vi "FL_Preprocess_and_save_incrementally.vi"(0 "Temporary file output path":path, 1 "Loop iteration":i32, 2 "Mouse face dir. swap":bool, 3 "Loop speed in ms":u16, 4 "Save every N seconds":u32=15, 5 "error in (no error)":errorcluster, 6 "Filter type":u16(ring)=5 items=["None", "Kalman 0.50", "Kalman 0.30", "Kalman 0.12", "Savitzky-Golay 3/5", "Savitzky-Golay 3/11", "Savitzky-Golay 3/31"], 7 "Sensor read input":T3(array[cluster]), 8 "Offset":sgl, 10 "Pixels per mm":dbl, 11 "Data flow controls in":T2, 12 "Diagram at recording bounds":T1, 13 "Sensor board size":string="Small") -> (14 "Eff. save interval":sgl, 15 "Latest sensor output (decoded)":string[][](array[string]), 16 "Fire TTL":bool, 17 "TTL out N":u8, 18 "Current TTL status":u8, 19 "error out":errorcluster)   [LabVIEW 2016]
uses:
  <vilib>/Utility/miscctls.llb/LVBoundsTypeDef.ctl
  SW_Globals.vi
  <vilib>/Utility/file.llb/Write Delimited Spreadsheet (string).vi
panel:
  in  "Max chunk size":i64=100000
  in  "Number of the file chunk":i32
  out "Chunk size (in bytes)":i64
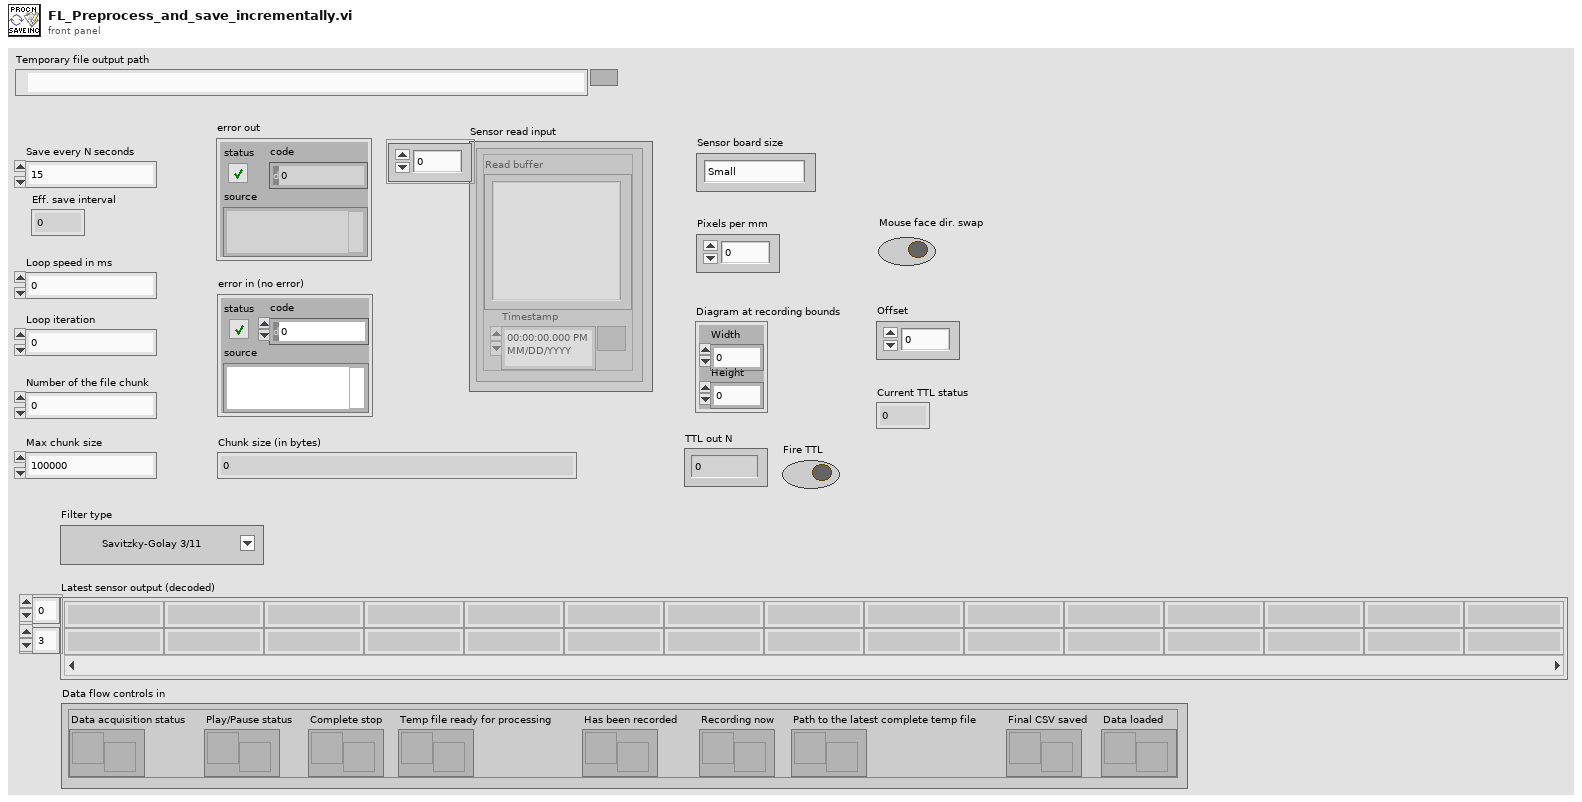
[diagram p1: front panel]
types:
  T1 = typedef "LVBoundsTypeDef.ctl" = cluster{"Width":u32, "Height":u32}
  T2 = cluster{"Data acquisition status":refnum<notifier>, "Play/Pause status":refnum<notifier>, "Complete stop":refnum<notifier>, "Temp file ready for processing":refnum<notifier>, "Has been recorded":refnum<notifier>, "Recording now":refnum<notifier>, "Path to the latest complete temp file":refnum<notifier>, "Final CSV saved":refnum<notifier>, "Data loaded":refnum<notifier>}
  T3 = cluster{"Read buffer":string, "Timestamp":timestamp}[]
  T4 = cluster{"ms since ON":u32, "delta time":u32, "X1":sgl, "Y1":sgl, "X2":sgl, "Y2":sgl, "TTL inputs":u8, "TTL outputs":u8, "Frame timestamp":timestamp, "Frame OK":bool}
  T5 = cluster{"X1 filtered":dbl, "Y1 filtered":dbl, "X2 filtered":dbl, "Y2 filtered":dbl, "X1 raw":dbl, "Y1 raw":dbl, "X2 raw":dbl, "Y2 raw":dbl}
  T6 = cluster{"R from center":dbl, "sin(a)":dbl, "Mouse Xc":dbl, "Mouse Yc":dbl, "X1-X2":dbl, "Y1-Y2":dbl, "Cage Xc":dbl, "Cage Yc":dbl}
  T7 = cluster{"R from center":dbl, "phi (mouse angular position in the cage)":dbl, "alpha (mouse rot. angle)":sgl, "X":dbl, "Y":dbl, "theta (from center towards mouse)":dbl, "beta (cage rot. against mouse)":sgl, "w (mouse angle to wall)":dbl}
  T8 = cluster{"Zone[1]":bool, "Zone[2]":bool, "Zone[3]":bool, "Zone[4]":bool, "Zone[5]":bool, "Zone[6]":bool, "Zone[7]":bool, "Zone[8]":bool, "Zone[9]":bool, "Zone[10]":bool, "Zone[11]":bool, "Zone[12]":bool, "Zone[13]":bool}
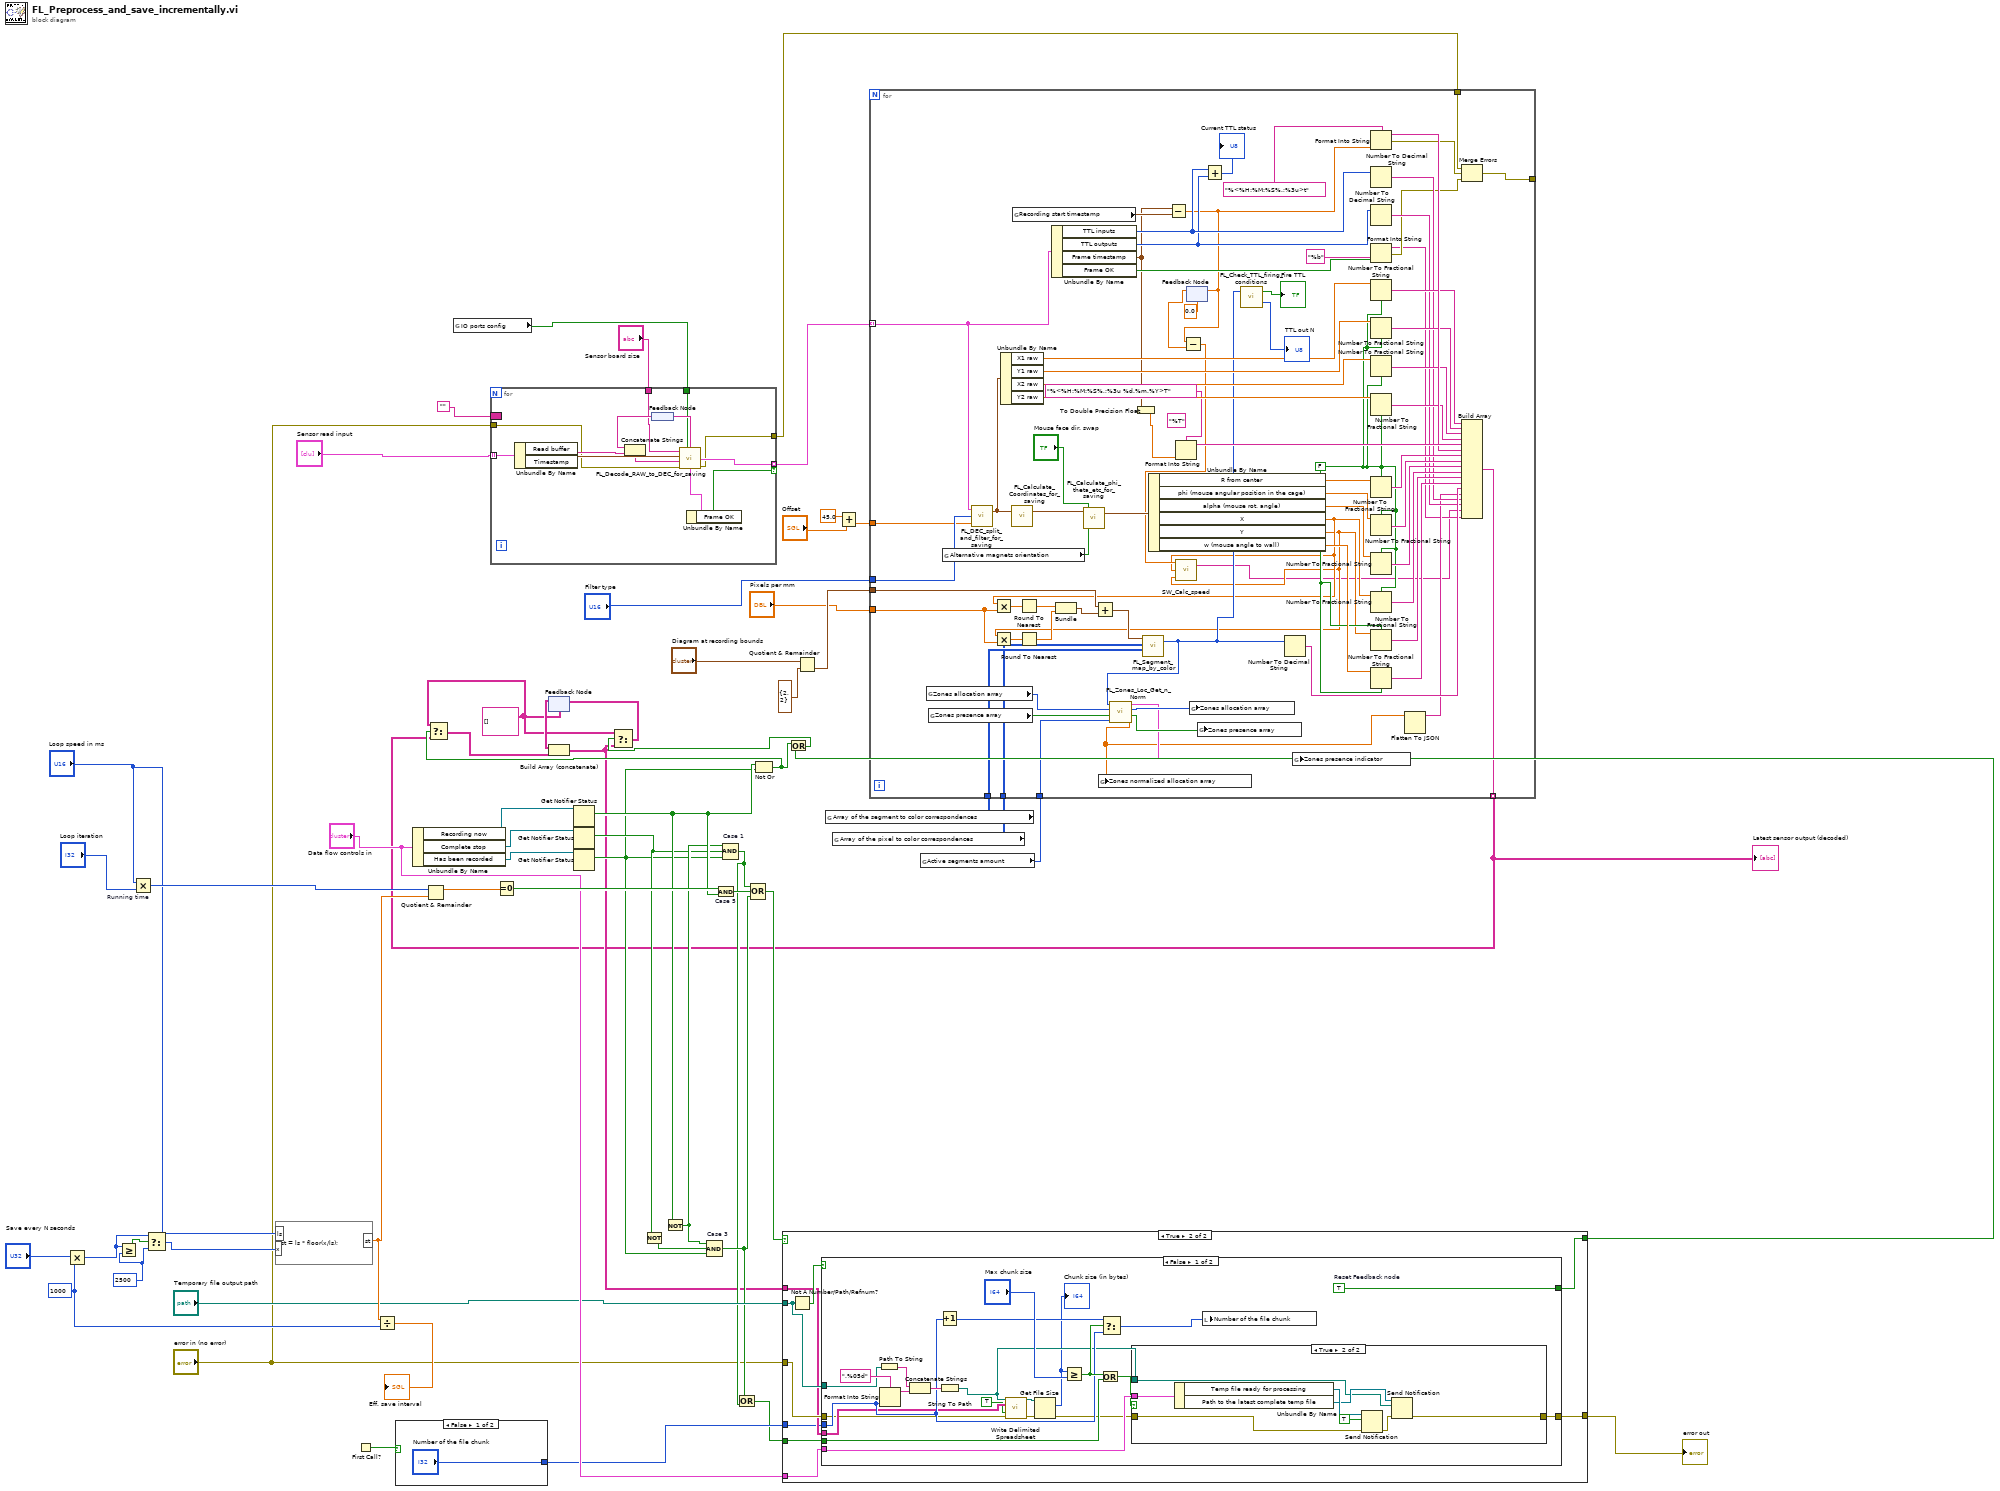
[diagram p0: block diagram]
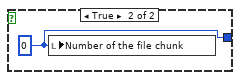
[diagram p2: hidden frame]
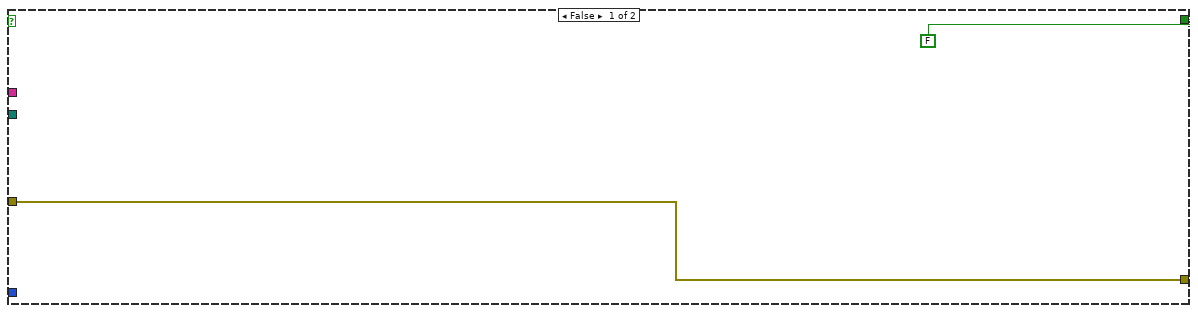
[diagram p3: hidden frame]
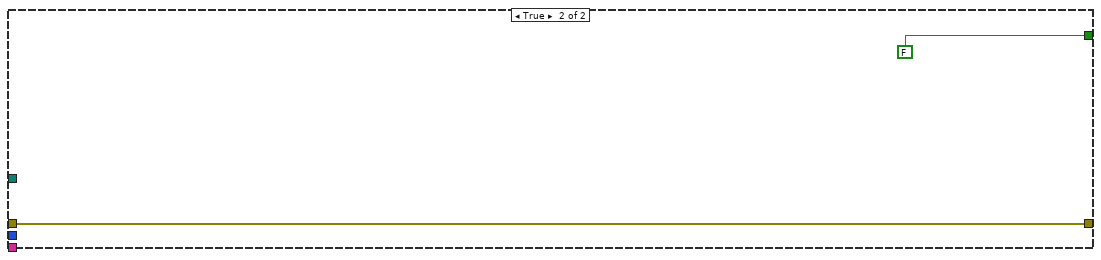
[diagram p5: hidden frame]
diagram:
  w31 = string[][] []
  w45 = u32 1000 ("y")
  w52 = 2500
  n1 = Multiply(x="Save every N seconds", y=w45) -> (x*y=w48:u32)
  n2 = Greater Or Equal?(x=w48, y=w52) -> (x >= y?=w53:bool)
  n3 = Multiply "Running time"(x="Loop speed in ms", y="Loop iteration") -> (x*y=w56:i32)
  n4 = Select(t=w48, s=w53, f=w52) -> (s? t:f=w50:u32)
  n5 = formula code="st = ls * floor(x/ls);"("ls"="Loop speed in ms", "x"=w50) -> ("st"=w47:dbl)
  n6 = First Call?() -> (First Call?: T/F=w40:bool)
  n7 = Divide(x=w47, y=w45) -> (x/y=→"Eff. save interval":dbl)
  n8 = case shown="False" w40 {
    tunnel: ["Number of the file chunk" w60] -> w34
    frame False {
    }
    frame True {
      w60 = 0 ("Number of the file chunk")
      n9 = local write "Number of the file chunk"(w60) -> ()
    }
  }
  n10 = Unbundle By Name("Data flow controls in") -> ("Recording now"=w39:refnum<notifier>, "Complete stop"=w38:refnum<notifier>, "Has been recorded"=w37:refnum<notifier>)
  n11 = Quotient & Remainder(x=w56, y=w47) -> (x-y*floor(x/y)=w54:dbl)  [unwired: 1 out]
  n12 = global read "SW_Globals.vi" "IO ports config"() -> (w1:bool[])
  n13 = for {
    tunnel: "Sensor read input" -> [w72] mode=indexing
    border: "" -> [_]
    tunnel: [w67] -> w18 mode=indexing if=w66
    tunnel: [w64] -> w19
    tunnel: "error in (no error)" -> [w63]
    tunnel: "Sensor board size" -> [w62]
    tunnel: w1 -> [w61]
    n14 = Unbundle By Name(w72) -> ("Read buffer"=w65:string, "Timestamp"=w71:timestamp)
    n15 = feedback #1() -> (w68:string)
    n16 = Concatenate Strings(w68, w65) -> (w70:string)
    n17 = call "FL_Decode_RAW_to_DEC_for_saving.vi"("Sensor board size"=w62, "IO ports config"=w61, "Input timestamp"=w71, "Input string"=w70, "Error In"=w63) -> ("Output string leftover"=w69:string, "DEC output cluster"=w67:T4, "Error Out"=w64:errorcluster)  [unwired: 1 in]
    n18 = feedback-in #1(w69) -> ()
    n19 = Unbundle By Name(w67) -> ("Frame OK"=w66:bool)
  }
  n20 = Equal To 0?(x=w54) -> (x = 0?=w55:bool)
  n21 = feedback #2(w31) -> (w43:string[][])
  n22 = Get Notifier Status(notifier=w39) -> (current notification=w28:bool)  [unwired: 1 in, 4 out]
  n23 = Get Notifier Status(notifier=w38) -> (current notification=w26:bool)  [unwired: 1 in, 4 out]
  n24 = Get Notifier Status(notifier=w37) -> (current notification=w25:bool)  [unwired: 1 in, 4 out]
  n25 = Not(x=w26) -> (.not. x?=w24:bool)
  n26 = Not(x=w28) -> (.not. x?=w27:bool)
  n27 = Compound Arithmetic op=AND "Case 3"(w27, w24, w25) -> (w33:bool)
  n28 = And "Case 5"(x=w55, y=w28) -> (x .and. y?=w58:bool)
  n29 = Compound Arithmetic op=AND "Case 1"(w27, w26, w25) -> (w22:bool)
  n30 = Or(x=w33, y=w22) -> (x .or. y?=w23:bool)
  n31 = Compound Arithmetic op=OR(w22, w58, w33) -> (w44:bool)
  n32 = Not Or(1:w25, 2:w28) -> (0:w30:bool)
  n33 = Quotient & Remainder(x="Diagram at recording bounds", y=T1 {"Width"=2, "Height"=2}) -> (floor(x/y)=w10:T1)  [unwired: 1 out]
  n34 = global read "SW_Globals.vi" "Array of the segment to color correspondences"() -> (w8:u32[][])
  n35 = global read "SW_Globals.vi" "Array of the pixel to color correspondences"() -> (w7:u32[][])
  n36 = Add(x=sgl 45.0, y="Offset") -> (x+y=w3:sgl)
  n37 = global read "SW_Globals.vi" "Active segments amount"() -> (w5:u8)
  n38 = for {
    tunnel: w18 -> [w146] mode=indexing
    tunnel: [w118] -> _
    tunnel: w19 -> [w117]
    tunnel: [w116] -> w16 mode=indexing
    tunnel: "Filter type" -> [w115]
    tunnel: w10 -> [w108]
    tunnel: "Pixels per mm" -> [w114]
    tunnel: w8 -> [w106]
    tunnel: w7 -> [w105]
    tunnel: w5 -> [w101]
    tunnel: w3 -> [w92]
    w120 = FALSE ("use system decimal point (T)")
    (unwired) "%T" ("format string")
    n39 = global read "SW_Globals.vi" "Zones allocation array"() -> (w102:i32[])
    n40 = global read "SW_Globals.vi" "Zones presence array"() -> (w100:bool[])
    n41 = global read "SW_Globals.vi" "Alternative magnets orientation"() -> (w73:bool)
    n42 = call "FL_DEC_split_and_filter_for_saving.vi"("Offset"=w92, "Filter type"=w115, "DEC input cluster"=w146) -> ("Magnets coords"=w148:T5)  [unwired: 1 in]
    n43 = Unbundle By Name(w148) -> ("X1 raw"=w138:dbl, "Y1 raw"=w136:dbl, "X2 raw"=w134:dbl, "Y2 raw"=w131:dbl)
    n44 = call "FL_Calculate_Coordinates_for_saving.vi"("Magnets coords in"=w148) -> ("Output cluster of data"=w147:T6)  [unwired: 2 in]
    n45 = global read "SW_Globals.vi" "Recording start timestamp"() -> (w145:timestamp)
    n46 = Unbundle By Name(w146) -> ("TTL inputs"=w87:u8, "TTL outputs"=w86:u8, "Frame timestamp"=w76:timestamp, "Frame OK"=w143:bool)
    n47 = call "FL_Calculate_phi_theta_etc_for_saving.vi"("Use alternative magnets orientation"=w73, "Mouse face dir. swap"="Mouse face dir. swap", "Input cluster of data"=w147) -> ("Output data cluster"=w139:T7)  [unwired: 1 in]
    n48 = To Double Precision Float(number=w76) -> (double precision float=w75:dbl)
    n49 = Unbundle By Name(w139) -> ("R from center"=w130:dbl, "phi (mouse angular position in the cage)"=w128:dbl, "alpha (mouse rot. angle)"=w126:sgl, "X"=w79:dbl, "Y"=w78:dbl, "w (mouse angle to wall)"=w122:dbl)
    n50 = Multiply(x=w79, y=w114) -> (x*y=w113:dbl)
    n51 = Multiply(x=w78, y=w114) -> (x*y=w112:dbl)
    n52 = Round To Nearest(number=w113) -> (nearest integer value=w111:dbl)
    n53 = Round To Nearest(number=w112) -> (nearest integer value=w110:dbl)
    n54 = Bundle(w111, w110) -> (w109:cluster{dbl, dbl})  [unwired: 1 in]
    n55 = Add(x=w108, y=w109) -> (x+y=w107:cluster{dbl, dbl})
    n56 = call "FL_Segment_map_by_color.vi"("Array of the segment to color correspondences"=w106, "Array of the pixel to color correspondences"=w105, "Mouse abs. coordinates, pix"=w107) -> ("Current segment' number"=w90:u32)  [unwired: 1 in, 1 out]
    n57 = call "FL_Zones_Loc_Get_n_Norm.vi"("Amount of active segments"=w101, "Zones presence array in"=w100, "Zones allocation array in"=w102, "Current segment' number"=w90) -> ("Zones normalized allocation array out"=w93:dbl[], "Zones presence array out"=w98:bool[], "Zones allocation array out"=w99:i32[], "Zones presence indicator cluster out"=w97:T8)  [unwired: 4 in]
    n58 = global write "SW_Globals.vi" "Zones normalized allocation array"(w93) -> ()
    n59 = Subtract(x=w76, y=w145) -> (x-y=w82:dbl)
    n60 = Format Into String(format string="%<%H:%M:%S%,;%3u %d.%m.%Y>T", w75) -> (resulting string=w141:string)  [unwired: 2 in, 1 out]
    n61 = feedback-in #3(w82) -> ()
    n62 = feedback #3(0.0) -> (w83:dbl)
    n63 = Subtract(x=w82, y=w83) -> (x-y=w80:dbl)
    n64 = call "SW_Calc_speed.vi"("Y coord, mm"=w78, "X coord, mm"=w79, "Time per frame, s"=w80) -> ("Mouse speed, mm/s"=w77:string)  [unwired: 1 out]
    n65 = global write "SW_Globals.vi" "Zones allocation array"(w99) -> ()
    n66 = global write "SW_Globals.vi" "Zones presence array"(w98) -> ()
    n67 = Add(x=w87, y=w86) -> (x+y=→"Current TTL status":u8)
    n68 = call "FL_Check_TTL_firing_conditions.vi"("Current segment' number (last value)"=w90) -> ("TTL out N"=→"TTL out N":u8, "Fire TTL"=→"Fire TTL":bool)  [unwired: 1 in]
    n69 = Number To Decimal String(number=w90) -> (decimal integer string=w104:string)  [unwired: 1 in]
    n70 = global write "SW_Globals.vi" "Zones presence indicator"(w97) -> ()
    n71 = Format Into String(format string="%<%H:%M:%S%.;%3u>t", w82) -> (resulting string=w140:string, error out=w119:errorcluster)  [unwired: 2 in]
    n72 = Number To Decimal String(number=w87) -> (decimal integer string=w95:string)  [unwired: 1 in]
    n73 = Number To Decimal String(number=w86) -> (decimal integer string=w96:string)  [unwired: 1 in]
    n74 = Format Into String(format string="%b", w143) -> (resulting string=w81:string, error out=w91:errorcluster)  [unwired: 2 in]
    n75 = Number To Fractional String(use system decimal point (T)=w120, number=w138) -> (F-format string=w137:string)  [unwired: 2 in]
    n76 = Number To Fractional String(use system decimal point (T)=w120, number=w136) -> (F-format string=w135:string)  [unwired: 2 in]
    n77 = Number To Fractional String(use system decimal point (T)=w120, number=w134) -> (F-format string=w133:string)  [unwired: 2 in]
    n78 = Number To Fractional String(use system decimal point (T)=w120, number=w131) -> (F-format string=w132:string)  [unwired: 2 in]
    n79 = Number To Fractional String(use system decimal point (T)=w120, number=w130) -> (F-format string=w129:string)  [unwired: 2 in]
    n80 = Number To Fractional String(use system decimal point (T)=w120, number=w128) -> (F-format string=w127:string)  [unwired: 2 in]
    n81 = Number To Fractional String(use system decimal point (T)=w120, number=w126) -> (F-format string=w125:string)  [unwired: 2 in]
    n82 = Number To Fractional String(use system decimal point (T)=w120, number=w79) -> (F-format string=w124:string)  [unwired: 2 in]
    n83 = Number To Fractional String(use system decimal point (T)=w120, number=w78) -> (F-format string=w123:string)  [unwired: 2 in]
    n84 = Number To Fractional String(use system decimal point (T)=w120, number=w122) -> (F-format string=w121:string)  [unwired: 2 in]
    n85 = Flatten To JSON(anything=w93) -> (JSON string=w94:string)  [unwired: 2 in, 1 out]
    n86 = Merge Errors(w117, w119, w91) -> (w118:errorcluster)
    n87 = Build Array(w137, w135, w133, w132, w141, w140, w129, w127, w125, w124, w123, w121, w104, w94, w95, w96, w77, w81) -> (w116:string[])
  }
  "Latest sensor output (decoded)" <- w16
  n88 = Select(t=w31, s=w30, f=w16) -> (s? t:f=w32:string[][])
  n89 = Build Array (concatenate)(w43, w32) -> (w21:string[][])
  n90 = case shown="True" w44 {
    tunnel: "Temporary file output path" -> [_ w158]
    tunnel: [FALSE w157] -> w41
    tunnel: "error in (no error)" -> [w149 w156]
    tunnel: [w149 w155] -> w14
    tunnel: w21 -> [_ w154]
    tunnel: "Data flow controls in" -> [_ w153]
    tunnel: w34 -> [_ w152]
    tunnel: w23 -> [_ w151]
    frame False {
    }
    frame True {
      n91 = Not A Number/Path/Refnum?(number/path/refnum=w158) -> (NaN/Path/Refnum?=w159:bool)
      n92 = case shown="False" w159 {
        tunnel: w158 -> [w174 _]
        tunnel: [w165 FALSE] -> w157
        tunnel: w156 -> [w161 w192]
        tunnel: [w172 w192] -> w155
        tunnel: w154 -> [w167 _]
        tunnel: w152 -> [w169 _]
        tunnel: w153 -> [w179 _]
        tunnel: w151 -> [w170 _]
        frame False {
          w165 = TRUE  # Reset Feedback node
          n93 = Path To String(path=w174) -> (string=w176:string)
          n94 = Format Into String(format string=".%05d", w169) -> (resulting string=w177:string)  [unwired: 2 in, 1 out]
          n95 = Concatenate Strings(w176, w177) -> (w178:string)
          n96 = Increment(x=w169) -> (x+1=w181:i32)
          n97 = String To Path(string=w178) -> (path=w168:path)
          n98 = call-poly <vilib>:"Write Delimited Spreadsheet.vi"("file path (dialog if empty)"=w168, "2D data"=w167, "append to file? (new file:F)"=TRUE, "error in (no error)"=w161) -> ("new file path (Not A Path if cancelled)"=w164:path, "error out"=w163:errorcluster)  [unwired: 10 in]
          n99 = Get File Size(file=w164, error in=w163) -> (size (in bytes)=w160:i64, 0:w162:errorcluster)  [unwired: 1 out]
          "Chunk size (in bytes)" <- w160
          n100 = Greater Or Equal?(x=w160, y="Max chunk size") -> (x >= y?=w173:bool)
          n101 = Or(x=w173, y=w170) -> (x .or. y?=w171:bool)
          n102 = Select(t=w181, s=w173, f=w169) -> (s? t:f=w180:i32)
          n103 = case shown="True" w171 {
            tunnel: w179 -> [_ w191]
            tunnel: w168 -> [_ w185]
            tunnel: w162 -> [w183 w187]
            tunnel: [w183 w186] -> w172
            frame False {
            }
            frame True {
              n104 = Unbundle By Name(w191) -> ("Temp file ready for processing"=w190:refnum<notifier>, "Path to the latest complete temp file"=w189:refnum<notifier>)
              n105 = Send Notification(notification=TRUE, notifier=w190, error in (no error)=w187) -> (error out=w188:errorcluster)  [unwired: 1 out]
              n106 = Send Notification(notification=w185, notifier=w189, error in (no error)=w188) -> (error out=w186:errorcluster)  [unwired: 1 out]
            }
          }
          n107 = local write "Number of the file chunk"(w180) -> ()
        }
        frame True {
        }
      }
    }
  }
  "error out" <- w14
  n108 = Or(x=w30, y=w41) -> (x .or. y?=w29:bool)
  n109 = Select(t=w31, s=w29, f=w21) -> (s? t:f=w42:string[][])
  n110 = feedback-in #2(w42) -> ()
